vi "SetAalborgClient.vi"(10 "Requested Concentration (%)":dbl min=0.0 max=100.0 step=1.0 format="%.2f", 11 "Requested Flowrate (l/min)":dbl min=0.0 max=360.0 step=1.0 format="%.2f") -> (0 "ServerMessages":string, 1 "WatchChannel":string)   [LabVIEW 2016]
panel:
  in  "Temperature channel":string
  in  "Pressure channel":string
  in  "maxFlowrate (l/min)":dbl min=0.0 max=360.0 step=1.0 format="%.2f"
  in  "minFlowrate (l/min)":dbl min=0.0 max=360.0 step=1.0 format="%.2f"
  in  "Mode":T1(ring)
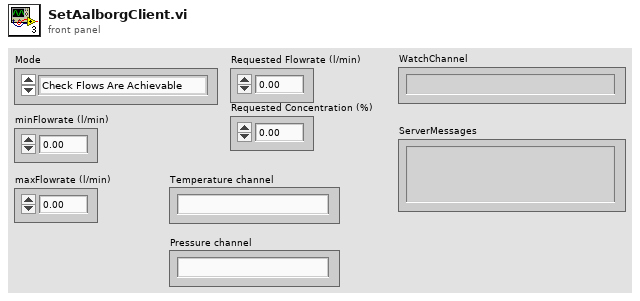
[diagram p1: front panel]
types:
  T1 = enum16{"Check Flows Are Achievable", "Set Flows"}
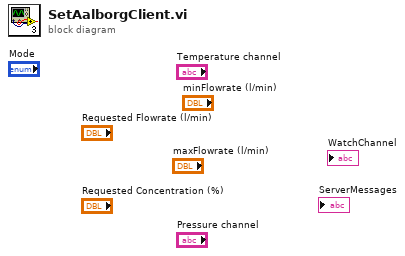
[diagram p0: block diagram]
diagram:
